vi "COMI INT Set Handler.vi"(6 "lParam":u32, 7 "nMessage":u32, 9 "Handler":u32, 10 "HandlerType":i32, 11 "hDevice":u32) -> (1 "Handler out":u32, 2 "function return":i32, 3 "hDevice out":u32, 4 "lParam out":u32)   [LabVIEW 2017, in "Comidll.lvlib"]
doc: "long (COMI_INT_SetHandler) (HANDLE hDevice, long HandlerType, HANDLE Handler, unsigned int nMessage, LPVOID lParam);"
uses:
  <userlib>/Comidll/Comidll.lvlib
  <userlib>/Comidll/Comidll.dll
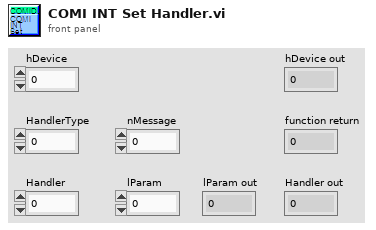
[diagram p1: front panel]
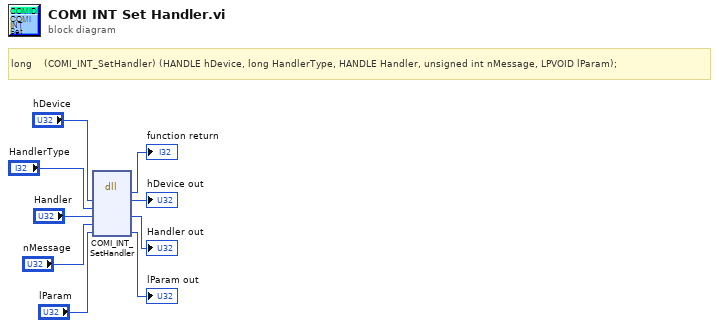
[diagram p0: block diagram]
diagram:
  # "long    (COMI_INT_SetHandler) (HANDLE hDevice, long HandlerType, HANDLE Handler, unsigned int nMessage, LPVOID lParam);"
  n1 = dll-call lib="C:/Program Files/National Instruments/LabVIEW 2017/user.lib/Comidll/Comidll.*" fn="COMI_INT_SetHandler"("hDevice"="hDevice", "HandlerType"="HandlerType", "Handler"="Handler", "nMessage"="nMessage", "lParam"="lParam") -> (→"function return":i32, "hDevice"=→"hDevice out":u32, "Handler"=→"Handler out":u32, "lParam"=→"lParam out":u32)  [unwired: 5 in, 2 out]
